vi "Copy Folder and Rename Files.vi"(8 "error in (no error)":errorcluster, 9 "File Name Suffix":string, 10 "Destination Folder":path, 11 "Source Folder":path) -> (0 "error out":errorcluster)   [LabVIEW 2014, in "SLL Application.lvlib"]
uses:
  SLL Application.lvlib
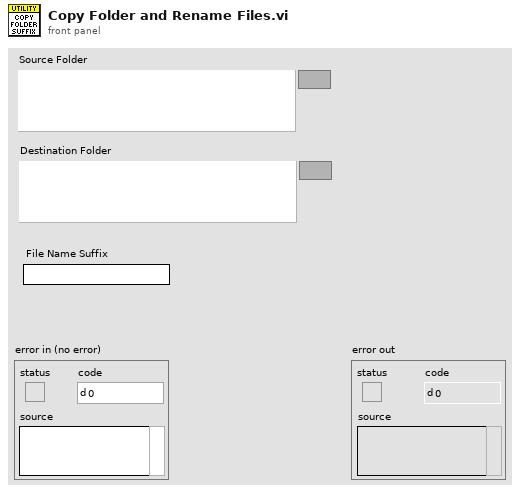
[diagram p1: front panel]
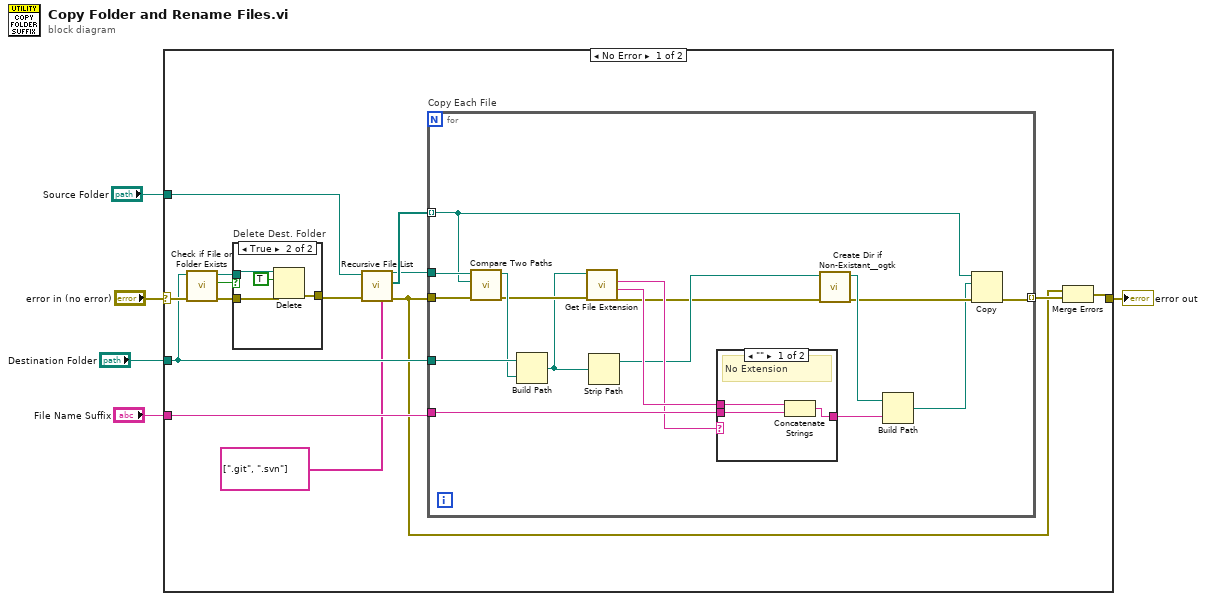
[diagram p0: block diagram]
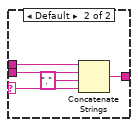
[diagram p3: hidden frame]
diagram:
  n1 = case shown="No Error" "error in (no error)" {
    selector: "error in (no error)" -> [w14 w50]
    tunnel: [w15 w50] -> w4
    tunnel: "Source Folder" -> [w18 _]
    tunnel: "Destination Folder" -> [w9 _]
    tunnel: "File Name Suffix" -> [w17 _]
    frame No Error {
      n2 = call <vilib>:"Check if File or Folder Exists.vi"("error in (no error)"=w14, "path"=w9) -> ("error out"=w13:errorcluster, "file or folder exists?"=w12:bool, "dup path"=w11:path)  [unwired: 7 in]
      n3 = case "Delete Dest. Folder" shown="True" w12 {
        tunnel: w13 -> [w20 w24]
        tunnel: w11 -> [_ w22]
        tunnel: [w20 w21] -> w10
        frame False {
        }
        frame True {
          n4 = Delete(path (use dialog)=w22, entire hierarchy (F)=TRUE, error in=w24) -> (error out=w21:errorcluster)  [unwired: 2 in, 2 out]
        }
      }
      n5 = call <vilib>:"Recursive File List.vi"("Folders to Exclude"=string[] [".git", ".svn"], "error in (no error)"=w10, "Folder Path"=w18) -> ("error out"=w6:errorcluster, "All Files in Dir"=w19:path[], "dup Folder Path"=w8:path)  [unwired: 4 in, 2 out]
      n6 = for "Copy Each File" {
        tunnel: w19 -> [w25] mode=indexing
        tunnel: w9 -> [w40]
        tunnel: w17 -> [w35]
        tunnel: w8 -> [w26]
        tunnel: w6 -> [w41]
        tunnel: [w28] -> w16 mode=indexing
        n7 = call <vilib>:"Compare Two Paths.vi"("error in (no error)"=w41, "Path 2"=w25, "Path 1"=w26) -> ("error out"=w38:errorcluster, "Relative Path from 1 to 2"=w39:path)  [unwired: 5 in, 2 out]
        n8 = Build Path(base path=w40, name or relative path=w39) -> (appended path=w37:path)
        n9 = call <vilib>:"Get File Extension.vi"("error in (no error)"=w38, "file"=w37) -> ("error out"=w32:errorcluster, "filename without extension"=w36:string, "lowercase file extension"=w34:string)  [unwired: 6 in, 1 out]
        n10 = Strip Path(path=w37) -> (stripped path=w33:path)  [unwired: 1 out]
        n11 = case shown="\"\"" w34 {
          selector: w34 -> [_ w46]
          tunnel: w36 -> [w44 w49]
          tunnel: w35 -> [w43 w48]
          tunnel: [w42 w45] -> w30
          frame "" {
            # "No Extension"
            n12 = Concatenate Strings(w44, w43) -> (w42:string)
          }
          frame Default {
            n13 = Concatenate Strings(w49, w48, "." ("string"), w46) -> (w45:string)
          }
        }
        n14 = call <userlib>:"Create Dir if Non-Existant__ogtk.vi"("error in (no error)"=w32, "Directory Path"=w33) -> ("error out"=w29:errorcluster, "dup Directory Path"=w31:path)  [unwired: 7 in, 1 out]
        n15 = Build Path(base path=w31, name or relative path=w30) -> (appended path=w27:path)
        n16 = Copy(8:w29, 10:w27, 11:w25) -> (0:w28:errorcluster)  [unwired: 2 in, 2 out]
      }
      n17 = Merge Errors(w6, w16) -> (w15:errorcluster)
    }
    frame Error {
    }
  }
  "error out" <- w4
